vi "readData.vi"(2 "Buffer Num":u8, 3 "SPI Config In":T1) -> (0 "Data Read":u8[](array[numeric]) format="%08b", 1 "SPI Config Out":T1)   [LabVIEW 2019]
uses:
  SPI/SPI Config.ctl
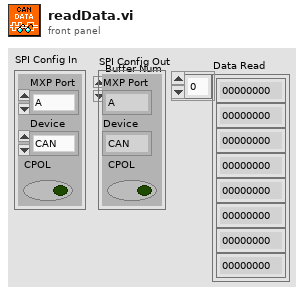
[diagram p1: front panel]
types:
  T1 = typedef "SPI Config.ctl" = cluster{"MXP Port":enum16{"A", "B"}, "Device":enum16{"CAN", "ENC", "IMU1", "IMU2"}, "CPOL":bool}
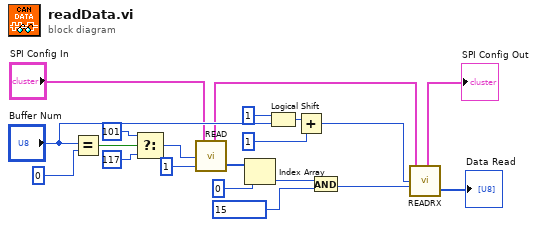
[diagram p0: block diagram]
diagram:
  n1 = Equal?(x="Buffer Num", y=u8 0) -> (x = y?=w19:bool)
  n2 = Select(t=u8 101, s=w19, f=u8 117 ("t")) -> (s? t:f=w9:u8)
  n3 = call "READ.vi"("Registers to Read"=u32 1, "Starting Address"=w9, "SPI Config In"="SPI Config In") -> ("Frames Read"=w7:u8[], "SPI Config Out"=w5:T1)
  n4 = Index Array(array=w7, index=0) -> (element=w15:u8)
  n5 = Logical Shift(y=i16 1, x="Buffer Num") -> (x << y=w11:u8)
  n6 = Add(x=w11, y=u8 1) -> (x+y=w1:u8)
  n7 = And(x=w15, y=u8 15) -> (x .and. y?=w2:u8)
  n8 = call "READRX.vi"("Registers to Read"=w2, "Reg. Select"=w1, "SPI Config In"=w5) -> ("Data Read"=→"Data Read":u8[], "SPI Config Out"=→"SPI Config Out":T1)
